vi "KITSAT_전체화면.vi"() -> ()   [LabVIEW 2011]
uses:
  <vilib>/Math Plots/3D Math Plots/3D Stem/3D Stem XCtrl/3D Stem.xctl
  <vilib>/Utility/file.llb/Write To Spreadsheet File (string).vi
  <vilib>/Math Plots/3D Math Plots/3D Stem/3D Stem Datatype/Public/Plot Helper (Vector).vi
  <vilib>/vision/NI_Vision_Development_Module.lvlib
  <vilib>/Math Plots/3D Math Plots/3D Stem/3D Stem Datatype/3D Stem Datatype.lvclass
panel:
  out "낙하 중 현재 위치":refnum<class "3D Plot Datatype.lvclass">[](xcontrol)
  in  "Stop 2":bool
  out "Boolean":bool
  out "공기 중 오염 농도":i32(graph)
  out "습 도":dbl(graph)
  out "Brightness Color (light temprature)":T1(plugin-control)
  out "Origin + Threshold":T1(plugin-control)
  in  "Image Type 5":T2 items=["Grayscale (U8)", "Grayscale (I16)", "Grayscale (SGL)", "Complex (CSG)", "RGB (U32)", "HSL (U32)", "RGB (U64)", "Grayscale (U16)"]
  out "Labeled Image (Threshold)":T1(plugin-control)
  in  "Connectivity":bool
  out "BCG (Brightness / Contrast / Gamma)":T1(plugin-control)
  in  "Image Type 2":T2 items=["Grayscale (U8)", "Grayscale (I16)", "Grayscale (SGL)", "Complex (CSG)", "RGB (U32)", "HSL (U32)", "RGB (U64)", "Grayscale (U16)"]
  in  "Stop":bool
  out "Original Image":T1(plugin-control)
  # "-KITSAT IMAGE PROCESSING PROGRAM-"
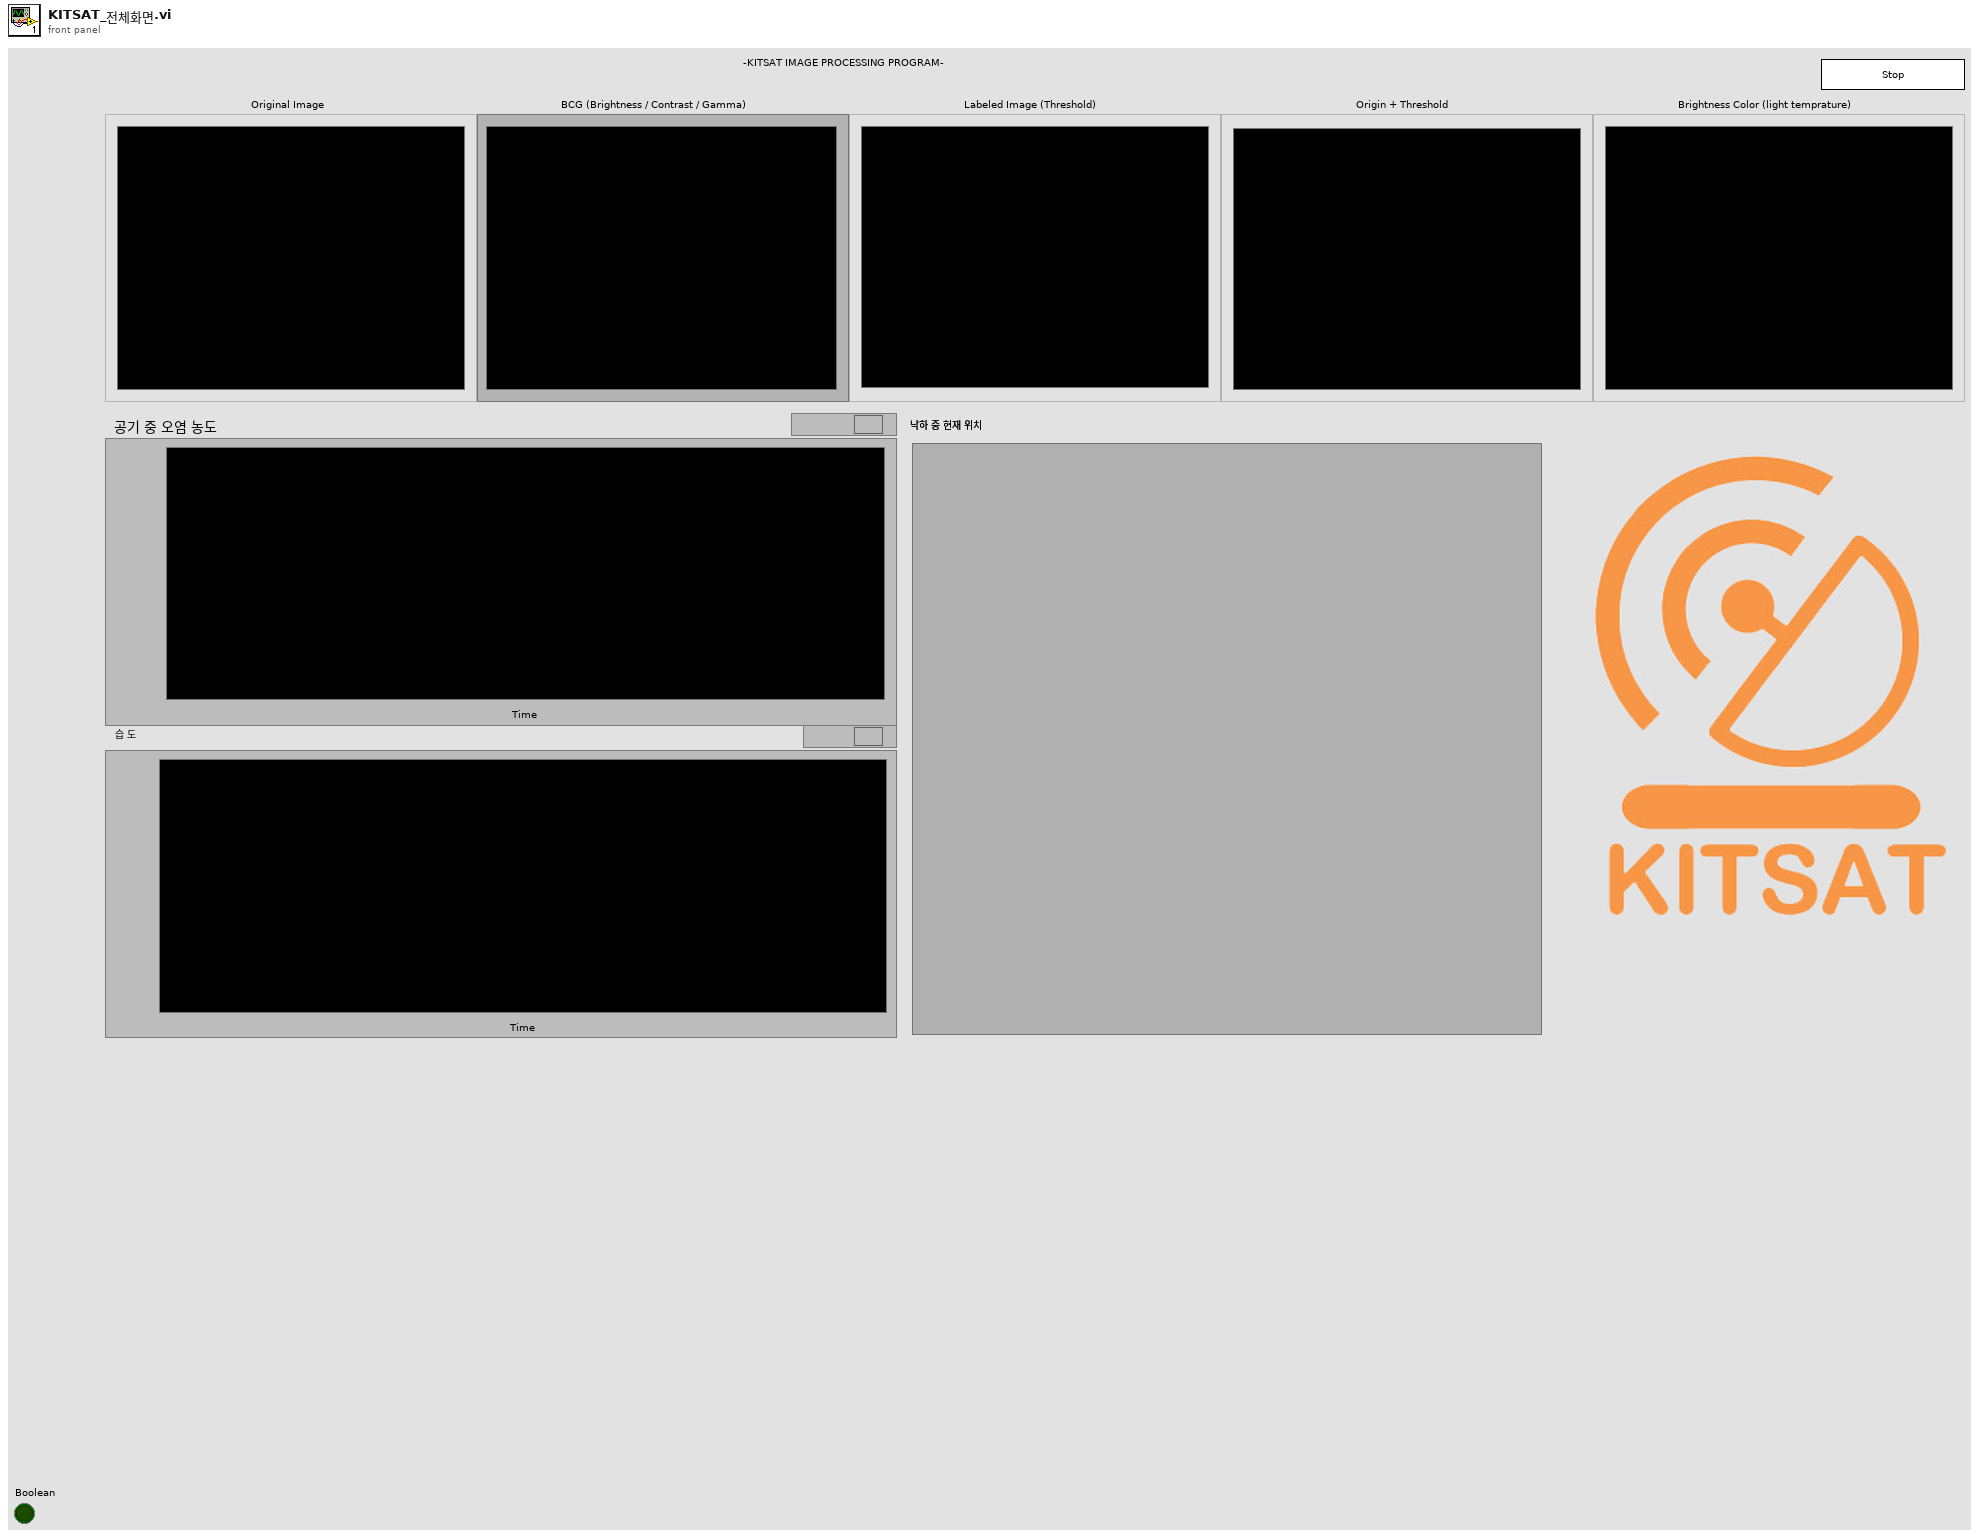
[diagram p1: front panel]
types:
  T1 = typedef "IMAQ Image.ctl" = refnum<image>
  T2 = typedef "Image Type" = u32
  T3 = typedef "AviRefnum.ctl" = refnum<k1>
  T4 = cluster{"Brightness":sgl, "Contrast":sgl, "Gamma":sgl}
  T5 = enum32{"AutoM", "Close", "Dilate", "Erode", "Gradient", "Gradient out", "Gradient in", "Hit miss", "Open", "PClose", "POpen", "Thick", "Thin"}
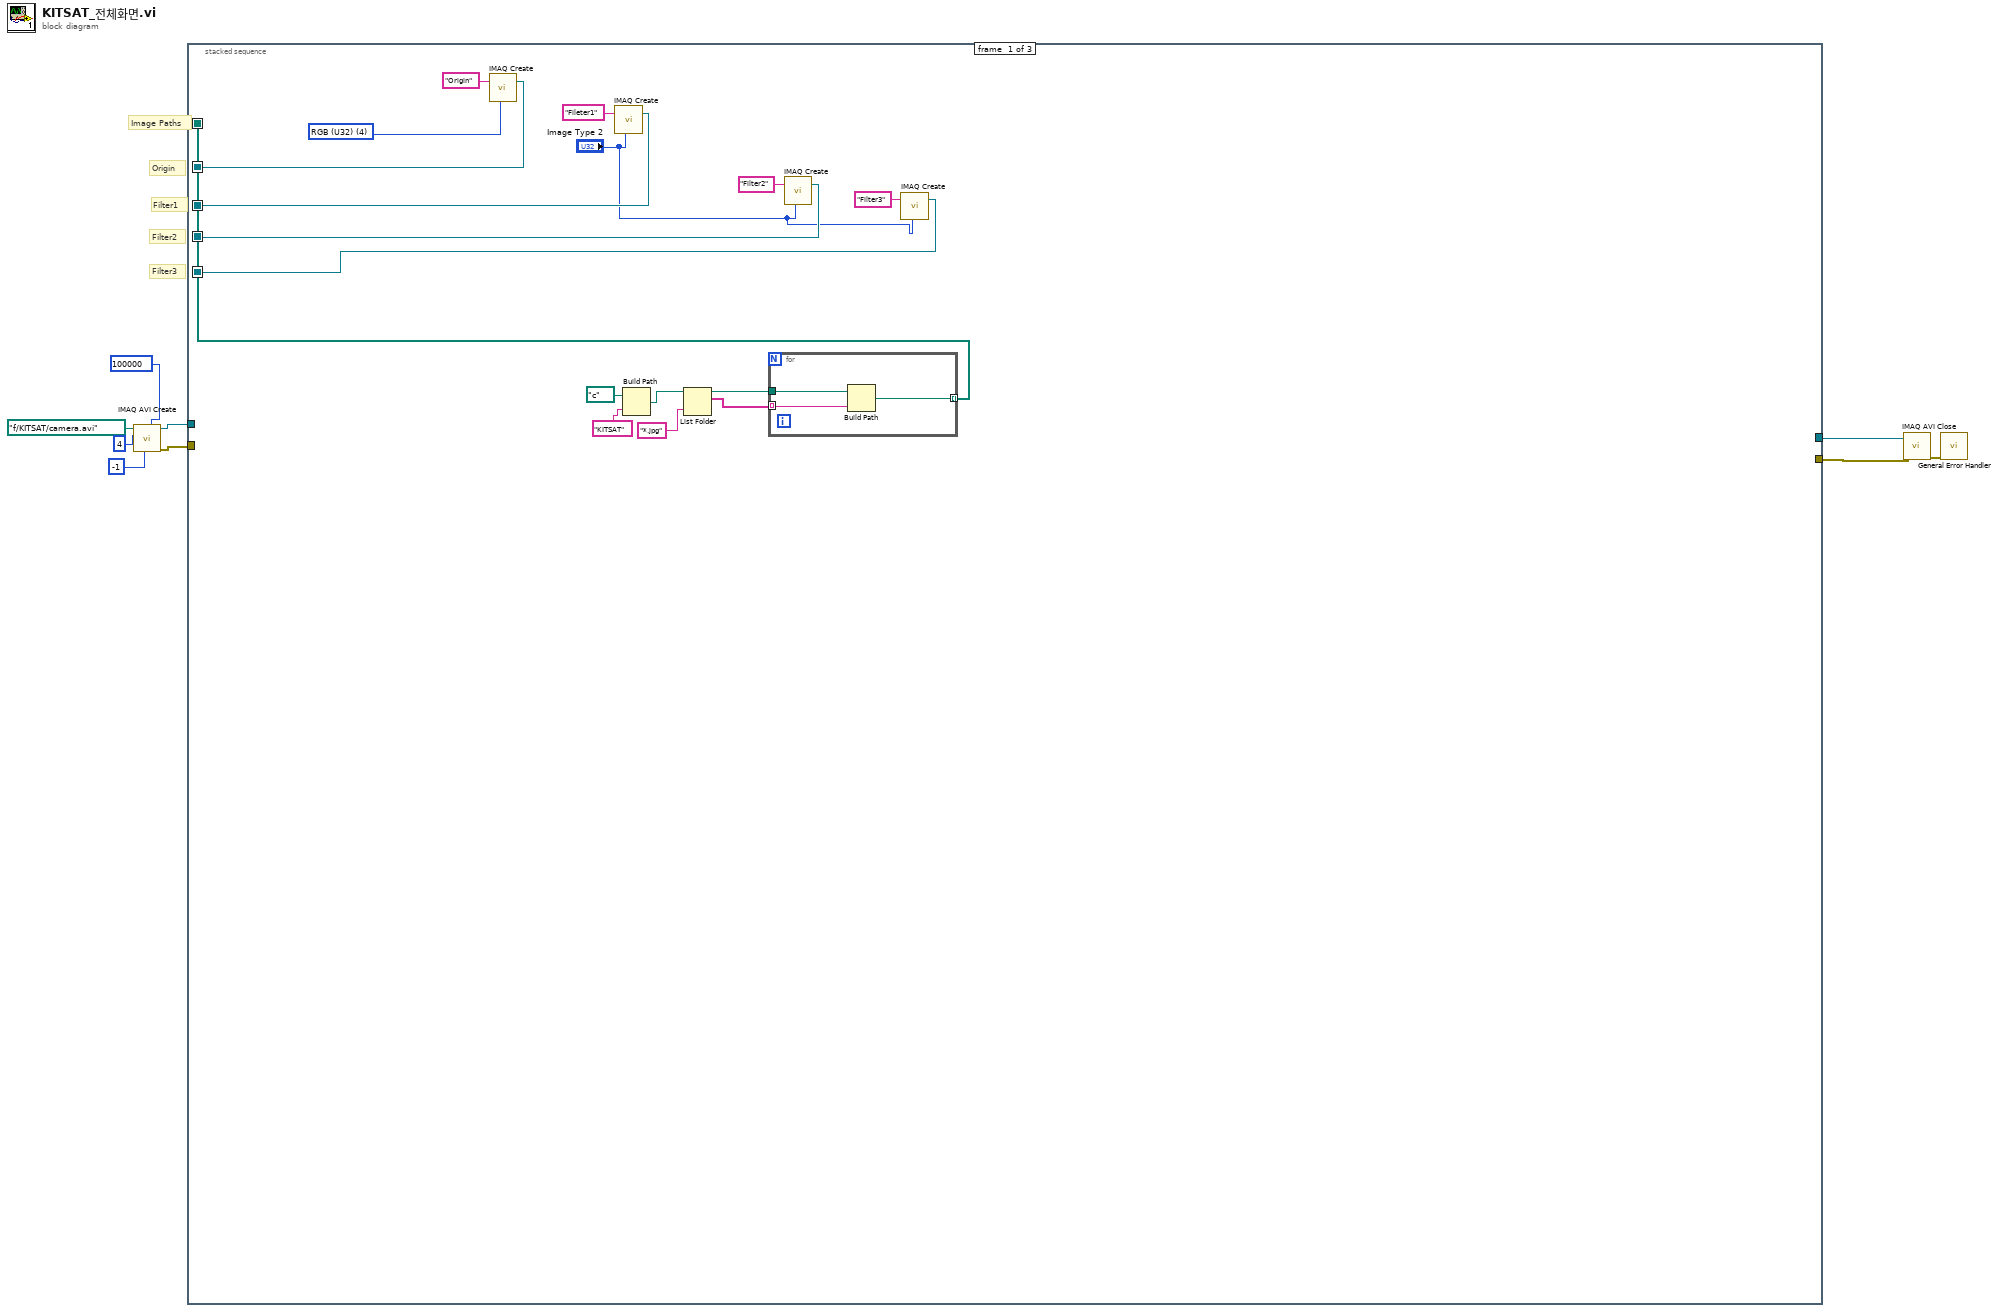
[diagram p0: block diagram]
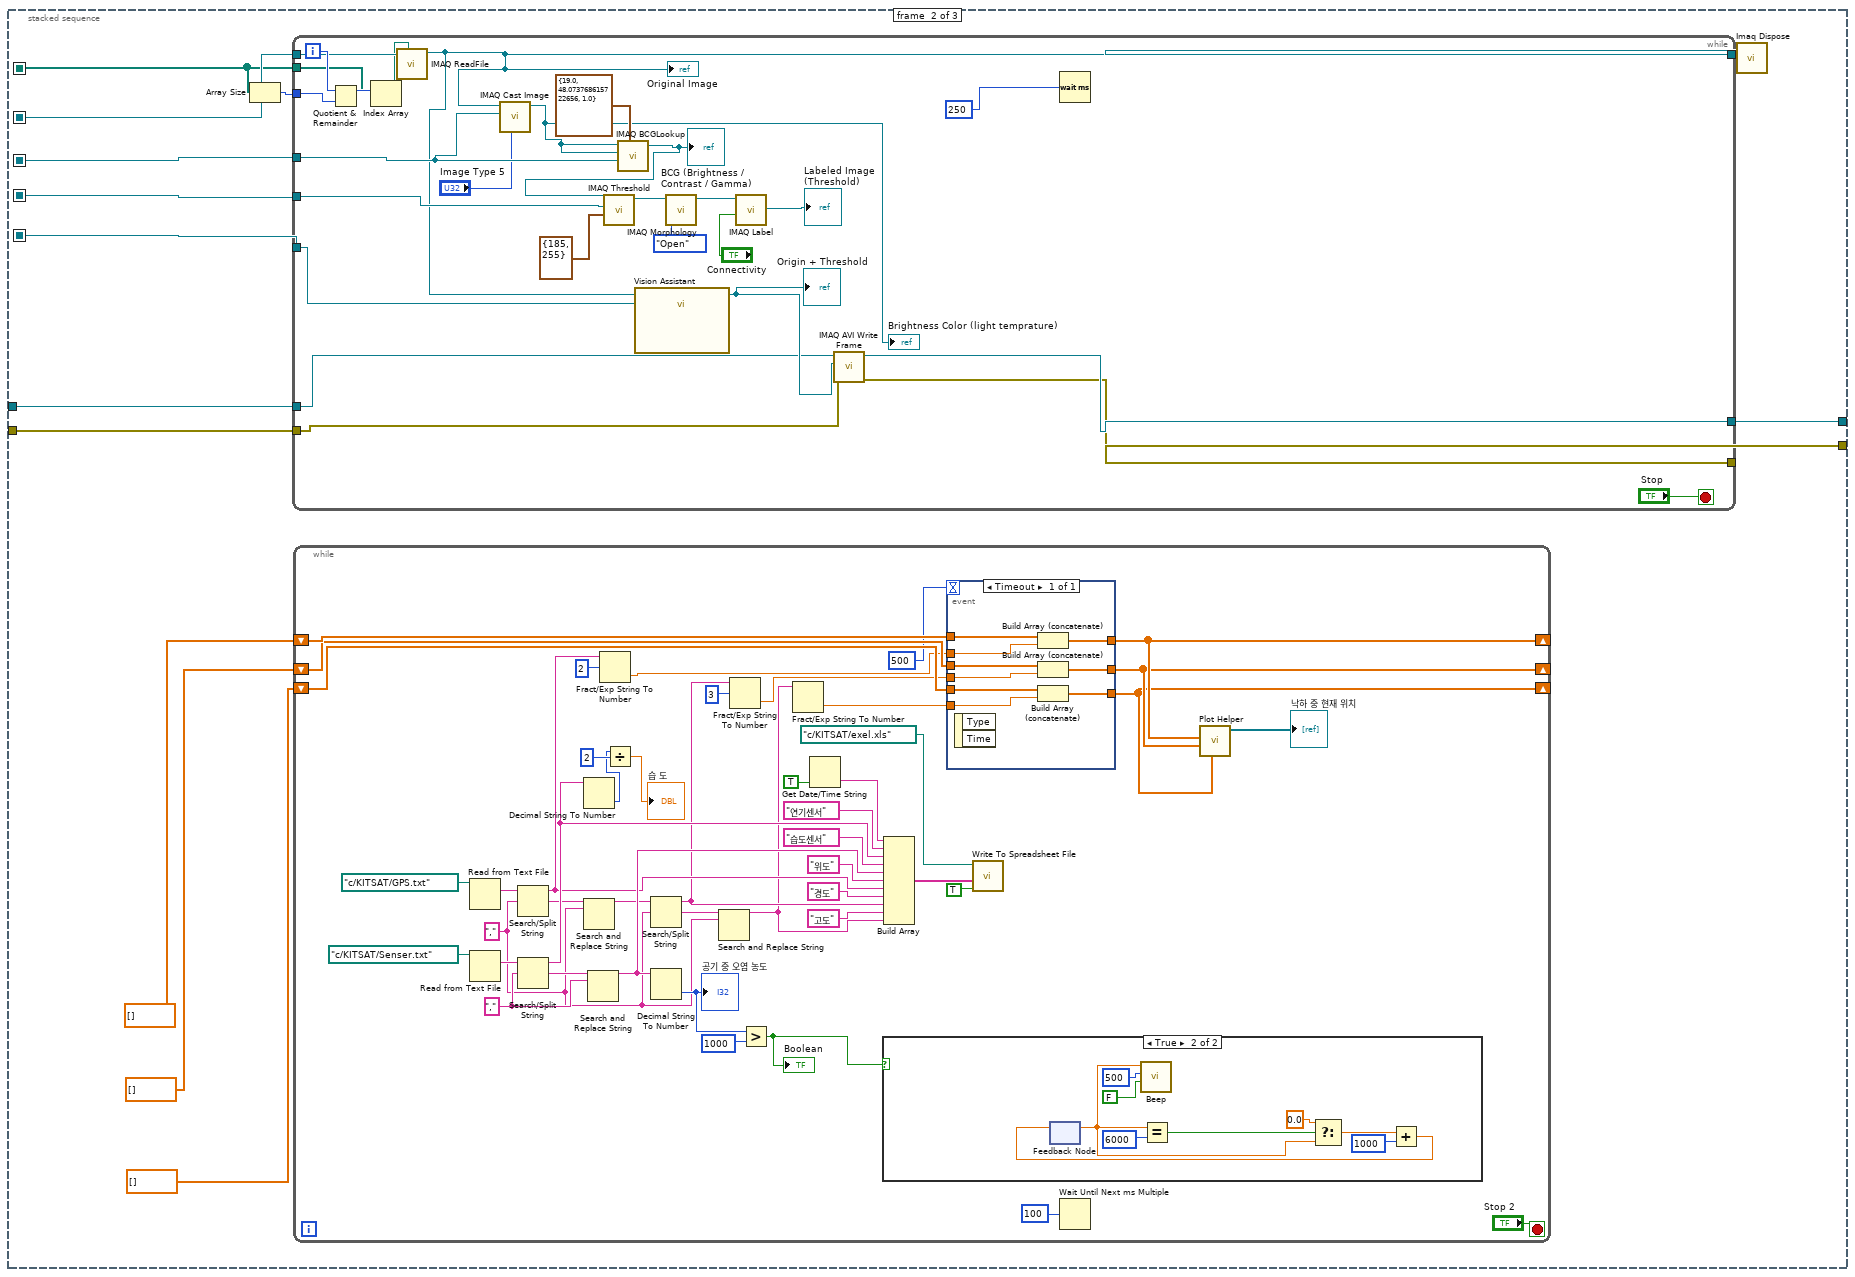
[diagram p2: hidden frame]
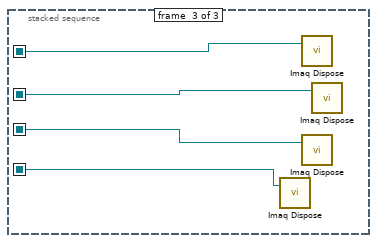
[diagram p4: hidden frame]
diagram:
  # "Filter3"
  # "Filter2"
  # "Filter1"
  # "Image Paths"
  # "Origin"
  n1 = call "IMAQ AVI Create"("Max Data Size"=u32 100000, "quality"=-1, "Frames Per Second"=u32 4, "AVI Path"=path "f:/KITSAT/camera.avi") -> ("error out"=w6:errorcluster, "Avi Refnum"=w7:T3)  [unwired: 6 in]
  n2 = stacked-sequence {
    seq-local: [w24 _ _] -> [_ w43 w138]
    seq-local: [w19 _ _] -> [_ w42 _]
    seq-local: [w15 _ _] -> [_ w40 w137]
    seq-local: [w14 _ _] -> [_ w39 w136]
    seq-local: [w12 _ _] -> [_ w38 w135]
    tunnel: w7 -> [_ w36 _]
    tunnel: [_ w35 _] -> w1
    tunnel: w6 -> [_ w34 _]
    tunnel: [_ w33 _] -> w2
    frame #0 {
      w10 = u32 4 items=["Grayscale(U8)", "Grayscale(I16)", "Grayscale(SGL)", "Complex(CSG)", "RGB (U32)", "HSL (U32)", "RGB (U64)", "Grayscale (U16)"] ("Image Type(RGB)")
      n3 = call "IMAQ Create"("Image Name"="Origin", "Image Type"=w10) -> ("New Image"=w24:T1)  [unwired: 2 in, 2 out]
      n4 = call "IMAQ Create"("Image Name"="Fileter1", "Image Type"="Image Type 2") -> ("New Image"=w15:T1)  [unwired: 2 in, 2 out]
      n5 = Build Path(base path=path "c:/", name or relative path="KITSAT") -> (appended path=w23:path)
      n6 = List Folder(path=w23, pattern="*.jpg") -> (path out=w22:path, filenames=w21:string[])  [unwired: 1 in, 3 out]
      n7 = for {
        tunnel: w21 -> [w28] mode=indexing
        tunnel: w22 -> [w29]
        tunnel: [w27] -> w19 mode=indexing
        n8 = Build Path(base path=w29, name or relative path=w28) -> (appended path=w27:path)
      }
      n9 = call "IMAQ Create"("Image Name"="Filter2", "Image Type"="Image Type 2") -> ("New Image"=w14:T1)  [unwired: 2 in, 2 out]
      n10 = call "IMAQ Create"("Image Name"="Filter3", "Image Type"="Image Type 2") -> ("New Image"=w12:T1)  [unwired: 2 in, 2 out]
    }
    frame #1 {
      n11 = Array Size(array=w42) -> (size(s)=w41:i32)
      n12 = while {
        tunnel: w43 -> [w130]
        tunnel: w42 -> [w131]
        tunnel: w41 -> [w133]
        tunnel: w40 -> [w118]
        tunnel: w39 -> [w121]
        tunnel: w38 -> [w116]
        tunnel: [w115] -> w37
        tunnel: w36 -> [w113]
        tunnel: [w112] -> w35
        tunnel: w34 -> [w111]
        tunnel: [w109] -> w33
        i -> [w134]
        stop <- "Stop" stop-if-true
        n13 = Quotient & Remainder(x=w134, y=w133) -> (x-y*floor(x/y)=w132:i32)  [unwired: 1 out]
        n14 = Index Array(array=w131, index=w132) -> (element=w129:path)
        n15 = call "IMAQ ReadFile"("File Path"=w129, "Image"=w130) -> ("Image Out"=w115:T1)  [unwired: 3 in, 6 out]
        "Original Image" <- w115
        n16 = call "IMAQ Cast Image"("Image Type"="Image Type 5", "Image Dst"=w118, "Image Src"=w115) -> ("Image Dst Out"=w110:T1)  [unwired: 7 in, 1 out]
        "Brightness Color (light temprature)" <- w110
        n17 = call "IMAQ BCGLookup"("Image Src"=w110, "BCG Values"=T4 {"Brightness"=19.0, "Contrast"=48.07377, "Gamma"=1.0}, "Image Mask"=w110, "Image Dst"=w118) -> ("Image Dst Out"=w122:T1)  [unwired: 3 in, 1 out]
        "BCG (Brightness / Contrast / Gamma)" <- w122
        n18 = call "IMAQ Threshold"("Range"=cluster{i32, i32} {185, 255} ("Threshold"), "Image Dst"=w121, "Image Src"=w122) -> ("Image Dst Out"=w125:T1)  [unwired: 3 in, 5 out]
        n19 = call "Vision Assistant"("Image In"=w115, "Image Dst"=w116) -> ("Image Out"=w114:T1)  [unwired: 24 in, 1 out]
        "Origin + Threshold" <- w114
        n20 = call "IMAQ Morphology"("Operation"=T5."Open", "Image Src"=w125) -> ("Image Dst Out"=w123:T1)  [unwired: 5 in, 4 out]
        n21 = call "IMAQ Label"("Connectivity 4/8 (8)"="Connectivity", "Image Src"=w123) -> ("Image Dst Out"=→"Labeled Image (Threshold)":T1)  [unwired: 2 in, 2 out]
        n22 = call "IMAQ AVI Write Frame"("error in (no error)"=w111, "Image"=w114, "Avi Refnum"=w113) -> ("error out"=w109:errorcluster, "Avi Refnum (duplicate)"=w112:T3)  [unwired: 7 in]
        n23 = Wait (ms)(milliseconds to wait=u32 250) -> ()  [unwired: 1 out]
      }
      n24 = while {
        shift-right: [w69] -> _
        shift-left: dbl[] [] -> [w73]
        shift-right: [w68] -> _
        shift-left: dbl[] [] -> [w72]
        shift-right: [w67] -> _
        shift-left: dbl[] [] -> [w71]
        stop <- "Stop 2" stop-if-true
        w61 = ","
        w74 = ","
        n25 = Read from Text File(file (use dialog)=path "c:/KITSAT/GPS.txt") -> (text=w66:string)  [unwired: 3 in, 3 out]
        n26 = Read from Text File(file (use dialog)=path "c:/KITSAT/Senser.txt") -> (text=w89:string)  [unwired: 3 in, 3 out]
        n27 = Search/Split String(string=w66, search string/char (-)=w61) -> (substring before match=w52:string, match + rest of string=w64:string)  [unwired: 1 in, 1 out]
        n28 = Search/Split String(string=w89, search string/char (-)=w74) -> (substring before match=w84:string, match + rest of string=w88:string)  [unwired: 1 in, 1 out]
        n29 = Decimal String To Number(string=w84) -> (number=w44:i32)  [unwired: 2 in, 1 out]
        n30 = Search and Replace String(input string=w64, search string=w61) -> (result string=w63:string)  [unwired: 6 in, 3 out]
        n31 = Search and Replace String(input string=w88, search string=w74) -> (result string=w79:string)  [unwired: 1 in, 8 out]
        n32 = Fract/Exp String To Number(string=w52, offset=2) -> (number=w58:dbl)  [unwired: 2 in, 1 out]
        n33 = Divide(x=w44, y=2) -> (x/y=→"습 도":dbl)
        n34 = Search/Split String(string=w63, search string/char (-)=w61) -> (substring before match=w50:string, match + rest of string=w62:string)  [unwired: 1 in, 1 out]
        n35 = Decimal String To Number(string=w79) -> (number=w87:i32)  [unwired: 2 in, 1 out]
        "공기 중 오염 농도" <- w87
        n36 = Search and Replace String(input string=w62, search string=w61) -> (result string=w48:string)  [unwired: 6 in, 3 out]
        n37 = Fract/Exp String To Number(string=w50, offset=3) -> (number=w57:dbl)  [unwired: 2 in, 1 out]
        n38 = Greater?(x=w87, y=1000) -> (0:w85:bool)
        "Boolean" <- w85
        n39 = Fract/Exp String To Number(string=w48) -> (number=w56:dbl)  [unwired: 3 in, 1 out]
        n40 = Get Date/Time String(want seconds? (F)=TRUE) -> (time string=w78:string)  [unwired: 2 in, 1 out]
        n41 = case shown="True" w85 {
          frame False {
          }
          frame True {
            n42 = feedback #1() -> (w100:dbl)  [unwired: 1 in]
            n43 = call <vilib>:"Beep.vi"("use system alert? (T)"=FALSE, "duration (msec)"=u32 500, "frequency (Hz)"=w100) -> ()  [unwired: 9 in]
            n44 = Equal?(x=w100, y=6000) -> (x = y?=w102:bool)
            n45 = Select(t=0.0, s=w102, f=w100) -> (s? t:f=w99:dbl)
            n46 = Add(x=w99, y=1000) -> (x+y=w105:dbl)
            n47 = feedback-in #1(w105) -> ()
          }
        }
        n48 = Build Array(w78, "연기센서", w84, "습도센서", w79, "위도" ("element"), w52, "경도" ("element"), w50, "고도" ("element"), w48) -> (w47:string[])
        n49 = event shown="[0] Timeout" {
          selector: _ -> [_]
          dyn-events: _ -> [_]
          timeout: 500 -> [_]
          tunnel: w73 -> [w98]
          tunnel: [w97] -> w69
          tunnel: w72 -> [w96]
          tunnel: [w95] -> w68
          tunnel: w71 -> [w94]
          tunnel: [w93] -> w67
          tunnel: w58 -> [w92]
          tunnel: w57 -> [w91]
          tunnel: w56 -> [w90]
          event Timeout {
            n50 = event-data() -> ()  [unwired: 1 in, 2 out]
            n51 = Build Array (concatenate)(w98, w92) -> (w97:dbl[])
            n52 = Build Array (concatenate)(w96, w91) -> (w95:dbl[])
            n53 = Build Array (concatenate)(w94, w90) -> (w93:dbl[])
          }
        }
        n54 = call-poly <vilib>:"Write To Spreadsheet File.vi"("append to file? (new file:F)"=TRUE, "1D data"=w47, "file path (dialog if empty)"=path "c:/KITSAT/exel.xls") -> ()  [unwired: 5 in, 1 out]
        n55 = Wait Until Next ms Multiple(millisecond multiple=u32 100 ("ms 배수")) -> ()  [unwired: 1 out]
        n56 = call-poly <vilib>:"Plot Helper.vi"("z vector"=w67, "y vector"=w68, "x vector"=w69) -> ("3D Plot lvclass Array out"=→"낙하 중 현재 위치":refnum<class "3D Plot Datatype.lvclass">[])  [unwired: 3 in, 5 out]
      }
      n57 = call "Imaq Dispose"("Image"=w37) -> ()  [unwired: 2 in, 4 out]
    }
    frame #2 {
      n58 = call "Imaq Dispose"("Image"=w135) -> ()  [unwired: 2 in, 4 out]
      n59 = call "Imaq Dispose"("Image"=w138) -> ()  [unwired: 2 in, 4 out]
      n60 = call "Imaq Dispose"("Image"=w136) -> ()  [unwired: 2 in, 4 out]
      n61 = call "Imaq Dispose"("Image"=w137) -> ()  [unwired: 2 in, 4 out]
    }
  }
  n62 = call "IMAQ AVI Close"("error in (no error)"=w2, "Avi Refnum"=w1) -> ("error out"=w5:errorcluster)  [unwired: 9 in]
  n63 = call <vilib>:"General Error Handler.vi"("error in (no error)"=w5) -> ()  [unwired: 10 in, 5 out]
